vi "DFD FIR Spectral Factorization.vi"(7 "method (Min-Max Phase)":enum16{"Min-Max Phase", "Linear Phase"}(ring), 8 "error in (no error)":errorcluster, 11 "H(n)":dbl[](array[numeric])) -> (0 "error out":errorcluster, 1 "H(n) 2":dbl[](array[numeric]), 2 "H(n) 1":dbl[](array[numeric]))   [LabVIEW 2017, in "NI_DigFilterLicensed.lvlib"]
doc: "Spectrally factorizes the <B>filter in</B> into two filters by specified method."
uses:
  <vilib>/addons/Digital Filter Design/NI_DigFilterLicensed.lvlib
  <vilib>/Analysis/2dsp.llb/1D Auto Correlation (DBL).vi
  <vilib>/addons/Digital Filter Design/_Misc.llb/dfd_Error Cluster From Error Code (Array).vi
  <vilib>/addons/Digital Filter Design/NI_DigFilter_Design.lvlib
  <vilib>/Analysis/NI_AALPro.lvlib
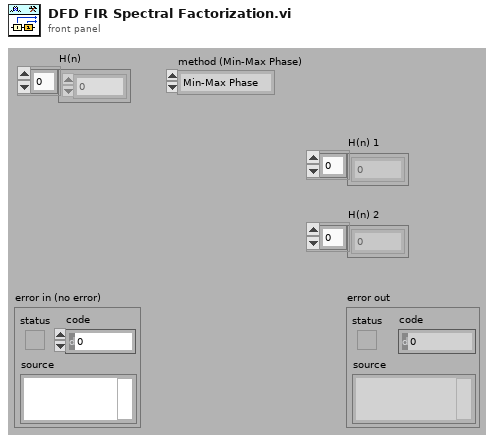
[diagram p1: front panel]
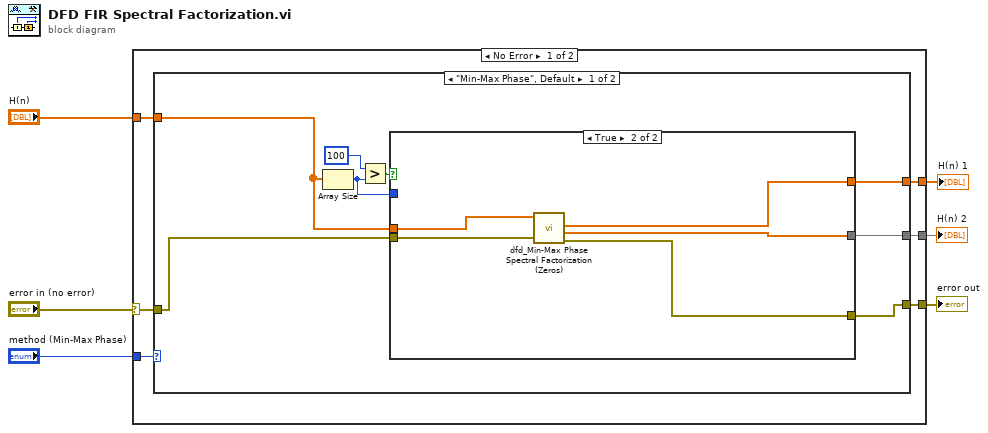
[diagram p0: block diagram]
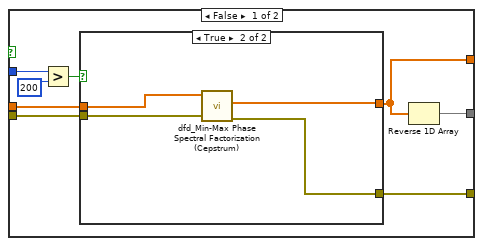
[diagram p2: hidden frame]
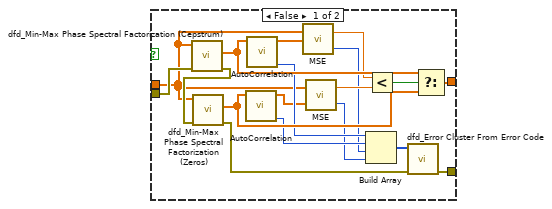
[diagram p3: hidden frame]
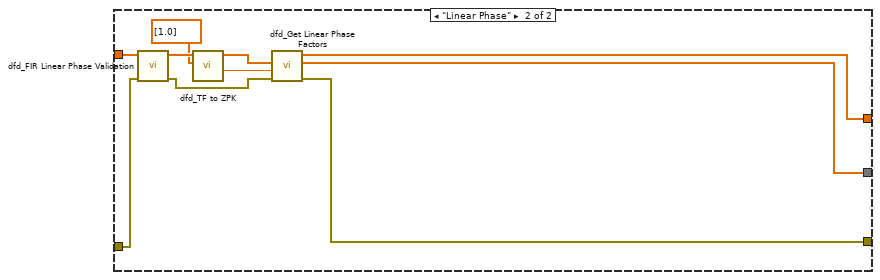
[diagram p4: hidden frame]
diagram:
  n1 = case shown="No Error" "error in (no error)" {
    selector: "error in (no error)" -> [w9 w66]
    tunnel: [w8 w66] -> w5
    tunnel: "H(n)" -> [w10 _]
    tunnel: [w12 _] -> w3
    tunnel: [w11 _] -> w2
    tunnel: "method (Min-Max Phase)" -> [w7 _]
    frame No Error {
      n2 = case shown="\"Min-Max Phase\", Default" w7 {
        tunnel: [w13 w59] -> w12
        tunnel: [w14 w58] -> w11
        tunnel: w10 -> [w16 w64]
        tunnel: w9 -> [w15 w63]
        tunnel: [w17 w65] -> w8
        frame "Min-Max Phase", Default {
          n3 = Array Size(array=w16) -> (size(s)=w18:i32)
          n4 = Greater?(x=100, y=w18) -> (0:w19:bool)
          n5 = case shown="True" w19 {
            tunnel: w16 -> [w28 w55]
            tunnel: w18 -> [w27 _]
            tunnel: w15 -> [w24 w54]
            tunnel: [w23 w53] -> w17
            tunnel: [w22 w52] -> w14
            tunnel: [w21 w51] -> w13
            frame False {
              n6 = Greater?(x=w27, y=200) -> (0:w25:bool)
              n7 = case shown="True" w25 {
                tunnel: w28 -> [w32 w50]
                tunnel: [w43 w49] -> w21
                tunnel: w24 -> [w42 w48]
                tunnel: [w36 w47] -> w23
                frame False {
                  n8 = call <vilib>:"dfd_Min-Max Phase Spectral Factorization (Cepstrum).vi"("error in (no error)"=w42, "numerator"=w32) -> ("error out"=w41:errorcluster, "minimum phase"=w45:dbl[])  [unwired: 8 out]
                  n9 = call <vilib>:"dfd_Min-Max Phase Spectral Factorization (Zeros).vi"("error in (no error)"=w41, "numerator"=w32) -> ("error out"=w37:errorcluster, "minimum phase"=w44:dbl[])  [unwired: 8 out]
                  n10 = call-poly <vilib>:"AutoCorrelation.vi"("X"=w44) -> ("error"=w39:i32, "Rxx"=w33:dbl[])  [unwired: 1 in, 8 out]
                  n11 = call-poly <vilib>:"AutoCorrelation.vi"("X"=w45) -> ("error"=w40:i32, "Rxx"=w35:dbl[])  [unwired: 1 in, 8 out]
                  n12 = call <vilib>:"MSE.vi"("X Values"=w35, "Y Values"=w32) -> ("error"=w30:i32, "mse"=w34:dbl)
                  n13 = call <vilib>:"MSE.vi"("X Values"=w33, "Y Values"=w32) -> ("error"=w29:i32, "mse"=w31:dbl)
                  n14 = Build Array(w40, w39, w30, w29) -> (w38:i32[])
                  n15 = Less?(x=w34, y=w31) -> (x < y?=w46:bool)
                  n16 = call-poly <vilib>:"dfd_Error Cluster From Error Code.vi"("error in (no error)"=w37, "error code (0)"=w38) -> ("error out"=w36:errorcluster)  [unwired: 9 out]
                  n17 = Select(t=w45, s=w46, f=w44) -> (s? t:f=w43:dbl[])
                }
                frame True {
                  n18 = call <vilib>:"dfd_Min-Max Phase Spectral Factorization (Cepstrum).vi"("error in (no error)"=w48, "numerator"=w50) -> ("error out"=w47:errorcluster, "minimum phase"=w49:dbl[])  [unwired: 8 out]
                }
              }
              n19 = Reverse 1D Array(array=w21) -> (reversed array=w22:dbl[])
            }
            frame True {
              n20 = call <vilib>:"dfd_Min-Max Phase Spectral Factorization (Zeros).vi"("error in (no error)"=w54, "numerator"=w55) -> ("error out"=w53:errorcluster, "maximum phase"=w52:dbl[], "minimum phase"=w51:dbl[])  [unwired: 7 out]
            }
          }
        }
        frame "Linear Phase" {
          n21 = call <vilib>:"dfd_FIR Linear Phase Validation.vi"("error in (no error)"=w63, "H(n) in"=w64) -> ("error out"=w60:errorcluster, "H(n) out"=w62:dbl[])  [unwired: 8 out]
          n22 = call <vilib>:"dfd_TF to ZPK.vi"("denominator"=dbl[] [1.0], "numerator"=w62) -> ("gain"=w57:dbl, "zeros"=w61:cdb[])  [unwired: 1 in, 7 out]
          n23 = call <vilib>:"dfd_Get Linear Phase Factors.vi"("error in (no error)"=w60, "gain"=w57, "zeros"=w61) -> ("error out"=w65:errorcluster, "H(n) 2"=w58:dbl[], "H(n) 1"=w59:dbl[])  [unwired: 2 in, 4 out]
        }
      }
    }
    frame Error {
    }
  }
  "error out" <- w5
  "H(n) 1" <- w3
  "H(n) 2" <- w2
